vi "Import VI Snippet.vi"(8 "error in (no error)":errorcluster, 9 "Drop Position":T1, 10 "VI Snippet (*.png)":path, 11 "VI Refnum (NaN=New VI)":refnum<vi>) -> (0 "error out":errorcluster, 1 "New VI?":bool, 3 "VI Refnum out":refnum<vi>)   [LabVIEW 2019]
doc: "Import a VI Snippet (*.png) image to the <b>VI Refnum</b> top level block diagram. If the <b>VI Refnum</b> is Not a Refnum this creates a new VI.\n\nCreated by: Ryan Pacini"
uses:
  <vilib>/Utility/miscctls.llb/LVPositionTypeDef.ctl
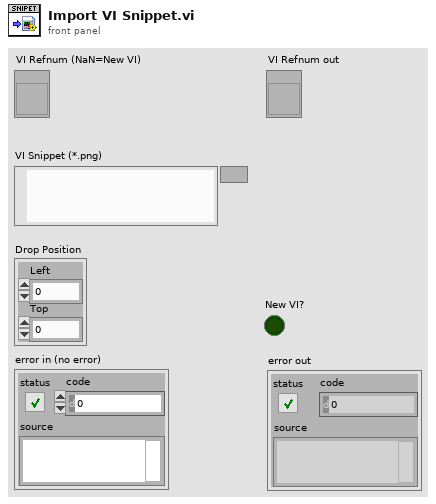
[diagram p1: front panel]
types:
  T1 = typedef "LVPositionTypeDef.ctl" = cluster{"Left":i32, "Top":i32}
  T2 = typedef "LVPointTypeDef.ctl" = cluster{"Horizontal":i16, "Vertical":i16}
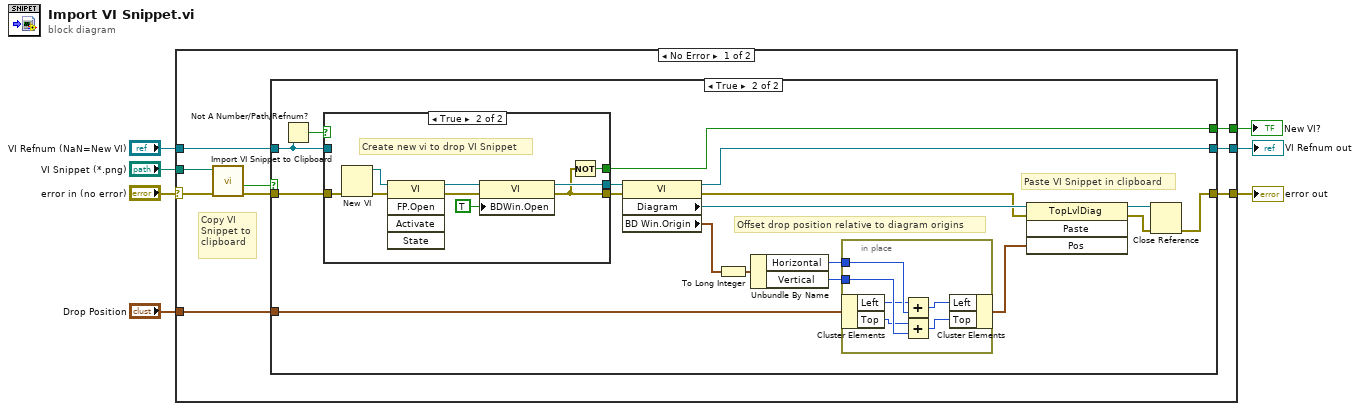
[diagram p0: block diagram]
diagram:
  n1 = case shown="No Error" "error in (no error)" {
    selector: "error in (no error)" -> [w16 w55]
    tunnel: "VI Snippet (*.png)" -> [w15 _]
    tunnel: "VI Refnum (NaN=New VI)" -> [w12 w54]
    tunnel: "Drop Position" -> [w11 _]
    tunnel: [w10 w55] -> w4
    tunnel: [w9 w54] -> w2
    tunnel: [w8 _] -> w1
    frame No Error {
      # "Copy VI\nSnippet to\nclipboard"
      n2 = call "Import VI Snippet to Clipboard.vi"("error in (no error)"=w16, "VI Snippet (*.png)"=w15) -> ("error out"=w14:errorcluster, "Copied to Clipboard?"=w13:bool)  [unwired: 8 in]
      n3 = case shown="True" w13 {
        tunnel: w14 -> [w18 w36]
        tunnel: w12 -> [w17 w21]
        tunnel: w11 -> [_ w35]
        tunnel: [w18 w34] -> w10
        tunnel: [w17 w33] -> w9
        tunnel: [_ w20] -> w8
        frame False {
          # "Failed to copy VI Snippet to clipboard"
        }
        frame True {
          # "Paste VI Snippet in clipboard"
          # "Offset drop position relative to diagram origins"
          n4 = Not A Number/Path/Refnum?(number/path/refnum=w21) -> (NaN/Path/Refnum?=w19:bool)
          n5 = case shown="True" w19 {
            tunnel: w36 -> [w43 w53]
            tunnel: [w44 w49] -> w23
            tunnel: [w43 w45] -> w22
            tunnel: w21 -> [w44 _]
            tunnel: [_ w46] -> w20
            frame False {
              # "Drop VI Snippet on VI Refnum specified"
            }
            frame True {
              # "Create new vi to drop VI Snippet"
              n6 = New VI(8:w53) -> (0:w52:errorcluster, 3:w51:refnum<vi>)  [unwired: 6 in]
              n7 = invoke class="VI" method="FP.Open"(reference=w51, error in=w52) -> (reference out=w50:refnum<vi>, error out=w48:errorcluster)  [unwired: 3 in, 3 out]
              n8 = property class="VI"(reference=w50, error in=w48, "BDWin.Open"=TRUE ("Block Diagram Window:Open")) -> (reference out=w49:refnum<vi>, error out=w45:errorcluster)
              n9 = Not(x=w45) -> (.not. x?=w46:bool)
            }
          }
          n10 = property class="VI"(reference=w23, error in=w22) -> (reference out=w33:refnum<vi>, error out=w29:errorcluster, "Diagram"=w30:refnum<vi>, "BD Win.Origin"=w28:T2)
          n11 = To Long Integer(number=w28) -> (32bit integer=w24:cluster{"Horizontal":i32, "Vertical":i32})
          n12 = Unbundle By Name(w24) -> ("Horizontal"=w27:i32, "Vertical"=w26:i32)
          n13 = in-place {
            in-place-border: w27 -> [w42]
            in-place-border: w26 -> [w41]
            n14 = in-place-cluster #1(w35) -> ("Left"=w40:i32, "Top"=w39:i32)
            n15 = Add(x=w40, y=w42) -> (x+y=w38:i32)
            n16 = Add(x=w39, y=w41) -> (x+y=w37:i32)
            n17 = in-place-cluster #1("Left"=w38, "Top"=w37) -> (w25:T1)
          }
          n18 = invoke class="TopLvlDiag" method="Paste"(reference=w30, error in=w29, "Pos"=w25) -> (reference out=w32:refnum<vi>, error out=w31:errorcluster)  [unwired: 1 in, 2 out]
          n19 = Close Reference(reference=w32, error in (no error)=w31) -> (error out=w34:errorcluster)
        }
      }
    }
    frame Error {
    }
  }
  "error out" <- w4
  "VI Refnum out" <- w2
  "New VI?" <- w1
